vi "updateQueue.vi"(9 "Waypoint Index":i32, 10 "new Waypoint":refnum<class "Waypoint.lvclass">, 11 "Waypoint Queue":refnum<queue>) -> (3 "queue out":refnum<queue>)   [LabVIEW 2013]
doc: "Change a single waypoint to a new waypoint"
uses:
  Logic/Classes/Waypoint/Waypoint.lvclass
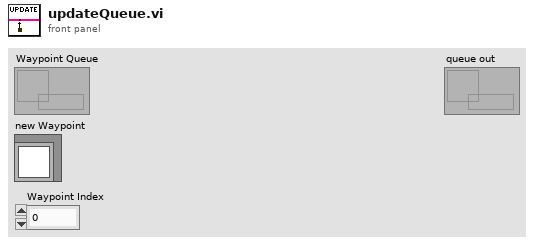
[diagram p1: front panel]
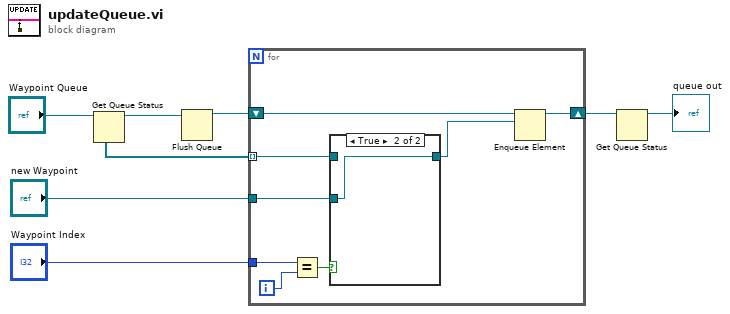
[diagram p0: block diagram]
diagram:
  n1 = Get Queue Status(queue="Waypoint Queue") -> (queue out=w7:refnum<queue>, elements=w6:refnum<class "Waypoint.lvclass">[])  [unwired: 2 in, 6 out]
  n2 = Flush Queue(queue=w7) -> (queue out=w4:refnum<queue>)  [unwired: 1 in, 2 out]
  n3 = for {
    tunnel: w6 -> [w11] mode=indexing
    shift-right: [w16] -> w5
    shift-left: w4 -> [w15]
    tunnel: "Waypoint Index" -> [w13]
    tunnel: "new Waypoint" -> [w9]
    i -> [w14]
    n4 = Equal?(x=w13, y=w14) -> (x = y?=w12:bool)
    n5 = case shown="True" w12 {
      tunnel: w11 -> [w17 _]
      tunnel: [w17 w18] -> w10
      tunnel: w9 -> [_ w18]
      frame False {
      }
      frame True {
      }
    }
    n6 = Enqueue Element(queue=w15, element=w10) -> (queue out=w16:refnum<queue>)  [unwired: 2 in, 2 out]
  }
  n7 = Get Queue Status(queue=w5) -> (queue out=→"queue out":refnum<queue>)  [unwired: 2 in, 7 out]
